vi "Compute Transform Matrix.vi"() -> (0 "Inverse Matrix":T2 format="%.3g", 1 "Beam Angle Deg":dbl[](array[numeric]), 2 "Calibration Factor m/s per MHz":dbl[](array[numeric]) format="%#.3f", 3 "Beam Separations":dbl[](array[numeric]) format="%#.3g", 4 "Meas Setup File":string, 5 "Fixed Axis":T1(ring))   [LabVIEW 2020]
uses:
  <vilib>/Analysis/Matrix/Datatypes/RealMatrix.ctl
  <vilib>/Analysis/baseanly.llb/Matrix Type of Inverse Matrix.ctl
  Globals/Meas_global.vi
  Globals/Constants_global.vi
  <vilib>/Analysis/baseanly.llb/Real Inverse Matrix.vi
  <vilib>/Analysis/NI_AALBase.lvlib
  <vilib>/Analysis/Matrix/NI_Matrix.lvlib
panel:
  out "Input array":dbl[][](array[numeric])
  out "Location when at Focal Point":dbl[](array[numeric])
  out "Beam Check Positions":dbl[][](array[numeric])
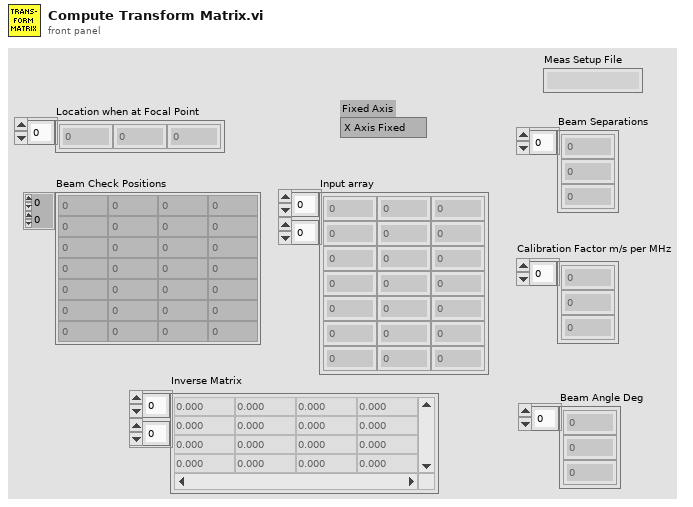
[diagram p1: front panel]
types:
  T1 = enum16{"X Axis Fixed", "Y Axis Fixed", "Z Axis Fixed"}
  T2 = typedef "NI_Matrix.lvlib/RealMatrix.ctl" = dbl[][]
  T3 = typedef "Post_Process.ctl" = enum16{"Take New Data", "Post Process Raw Data File"}
  T4 = typedef "NI_AALBase.lvlib/Matrix Type of Inverse Matrix.ctl" = enum32{"General", "Positive Definite", "Lower Triangular", "Upper Triangular"}
  T5 = typedef "Fixed Axis.ctl" = enum16{"X Axis Fixed", "Y Axis Fixed", "Z Axis Fixed"}
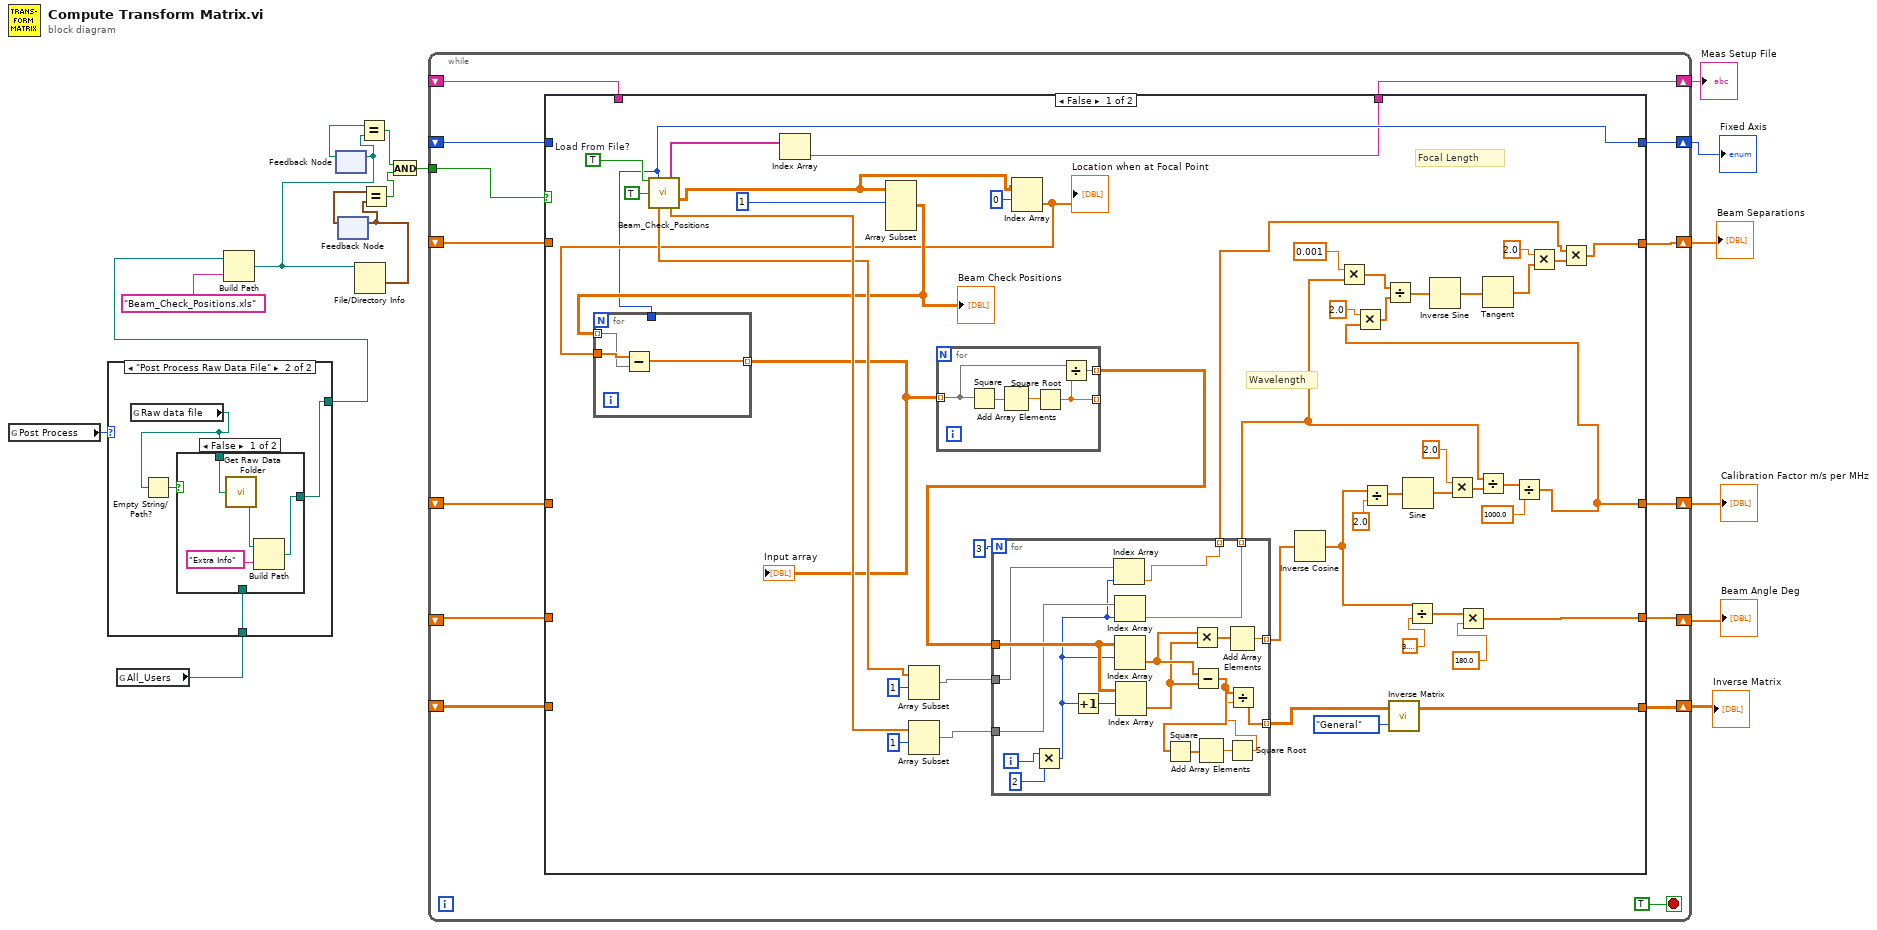
[diagram p0: block diagram]
diagram:
  n1 = global read "Meas_global.vi" "Post Process"() -> (w15:T3)
  n2 = global read "Constants_global.vi" "All_Users"() -> (w7:path)
  n3 = case shown="\"Post Process Raw Data File\"" w15 {
    tunnel: [w18 w22] -> w13
    tunnel: w7 -> [w18 w19]
    frame "Take New Data" {
    }
    frame "Post Process Raw Data File" {
      n4 = global read "Meas_global.vi" "Raw data file"() -> (w21:path)
      n5 = Empty String/Path?(string/path=w21) -> (empty?=w20:bool)
      n6 = case shown="False" w20 {
        tunnel: [w26 w27] -> w22
        tunnel: w21 -> [w24 _]
        tunnel: w19 -> [_ w27]
        frame False {
          n7 = call "Get Raw Data Folder.vi"("Raw data file"=w24) -> ("Main Raw Data Folder"=w23:path)
          n8 = Build Path(base path=w23, name or relative path="Extra Info") -> (appended path=w26:path)
        }
        frame True {
        }
      }
    }
  }
  n9 = Build Path(base path=w13, name or relative path="Beam_Check_Positions.xls" ("Substring")) -> (appended path=w5:path)
  n10 = feedback #1() -> (w4:path)  [unwired: 1 in]
  n11 = feedback-in #1(w5) -> ()
  n12 = feedback #2() -> (w17:timestamp)  [unwired: 1 in]
  n13 = File/Directory Info(path=w5) -> (last mod=w16:timestamp)  [unwired: 1 in, 6 out]
  n14 = feedback-in #2(w16) -> ()
  n15 = Equal?(x=w4, y=w5) -> (x = y?=w2:bool)
  n16 = Equal?(x=w17, y=w16) -> (x = y?=w3:bool)
  n17 = And(x=w2, y=w3) -> (x .and. y?=w1:bool)
  n18 = while {
    tunnel: w1 -> [w32]
    shift-right: [w40] -> w12
    shift-left: _ -> [w39]
    shift-right: [w36] -> w9
    shift-left: _ -> [w35]
    shift-right: [w37] -> w10
    shift-left: _ -> [w34]
    shift-right: [w38] -> w11
    shift-left: _ -> [w33]
    shift-right: [w31] -> w8
    shift-left: _ -> [w30]
    shift-right: [w29] -> w6
    shift-left: _ -> [w28]
    stop <- TRUE stop-if-true
    n19 = case shown="False" w32 {
      tunnel: [w89 w121] -> w40
      tunnel: w39 -> [_ w121]
      tunnel: [w50 w118] -> w38
      tunnel: [w49 w119] -> w37
      tunnel: [w48 w120] -> w36
      tunnel: w35 -> [_ w120]
      tunnel: w34 -> [_ w119]
      tunnel: w33 -> [_ w118]
      tunnel: [w44 w117] -> w31
      tunnel: w30 -> [_ w117]
      tunnel: [w42 w116] -> w29
      tunnel: w28 -> [_ w116]
      frame False {
        w80 = TRUE  # Load From File?
        # "Focal Length"
        # "Wavelength"
        n20 = call "Beam_Check_Positions.vi"("Load From File?"=w80, "Give Focal Point Info (F)"=TRUE) -> ("Fixed Axis"=w44:T5, "Setup File"=w43:string[], "Primary Beam Positions"=w77:dbl[][], "Focal Length"=w54:dbl[], "Wavelength (nm)"=w70:dbl[])  [unwired: 5 in, 4 out]
        n21 = Index Array(array=w43) -> (element=w42:string)  [unwired: 1 in]
        n22 = Array Subset(array=w77, index (row)=1 ("index")) -> (w47:dbl[][])  [unwired: 3 in]
        "Beam Check Positions" <- w47
        n23 = Array Subset(array=w54, index=1) -> (w53:dbl[])  [unwired: 1 in]
        n24 = Array Subset(array=w70, index=1) -> (w68:dbl[])  [unwired: 1 in]
        n25 = Index Array(array=w77, index (row)=0) -> (element=w46:dbl[])  [unwired: 1 in]
        "Location when at Focal Point" <- w46
        n26 = for {
          tunnel: w47 -> [w91] mode=indexing
          tunnel: w46 -> [w92]
          tunnel: w44 -> [_]
          tunnel: [w90] -> w45 mode=indexing
          n27 = Subtract(x=w92, y=w91) -> (x-y=w90:dbl[])
        }
        "Input array" <- w45
        n28 = for {
          tunnel: w45 -> [w112] mode=indexing
          tunnel: [w113] -> _ mode=indexing
          tunnel: [w111] -> w87 mode=indexing
          n29 = Square(x=w112) -> (x^2=w115:dbl[])
          n30 = Add Array Elements(numeric array=w115) -> (sum=w114:dbl)
          n31 = Square Root(x=w114) -> (sqrt(x)=w113:dbl)
          n32 = Divide(x=w112, y=w113) -> (x/y=w111:dbl[])
        }
        n33 = for {
          N: 3 -> [_]
          tunnel: w87 -> [w108]
          tunnel: [w105] -> w86 mode=indexing
          tunnel: [w100] -> w82 mode=indexing
          tunnel: w68 -> [w97]
          tunnel: [w96] -> w63 mode=indexing
          tunnel: w53 -> [w94]
          tunnel: [w93] -> w51 mode=indexing
          i -> [w110]
          n34 = Multiply(x=w110, y=2) -> (x*y=w95:i32)
          n35 = Increment(x=w95) -> (x+1=w107:i32)
          n36 = Index Array(array=w94, index=w95) -> (element=w93:dbl)
          n37 = Index Array(array=w97, index=w95) -> (element=w96:dbl)
          n38 = Index Array(array=w108, index (row)=w95) -> (element=w104:dbl[])  [unwired: 1 in]
          n39 = Index Array(array=w108, index (row)=w107) -> (element=w103:dbl[])  [unwired: 1 in]
          n40 = Multiply(x=w104, y=w103) -> (x*y=w106:dbl[])
          n41 = Subtract(x=w104, y=w103) -> (x-y=w99:dbl[])
          n42 = Square(x=w99) -> (x^2=w102:dbl[])
          n43 = Add Array Elements(numeric array=w102) -> (sum=w101:dbl)
          n44 = Add Array Elements(numeric array=w106) -> (sum=w105:dbl)
          n45 = Square Root(x=w101) -> (sqrt(x)=w98:dbl)
          n46 = Divide(x=w99, y=w98) -> (x/y=w100:dbl[])
        }
        n47 = Inverse Cosine(1:w86) -> (0:w75:dbl[])
        n48 = Multiply(x=0.001, y=w63) -> (x*y=w61:dbl[])
        n49 = Divide(x=w75, y=2.0) -> (x/y=w73:dbl[])
        n50 = call-poly <vilib>:"Inverse Matrix.vi"("matrix type"=Matrix_Type_of_Inverse_Matrix."General", "Input Matrix"=w82) -> ("Inverse Matrix"=w89:T2)  [unwired: 1 out]
        n51 = Sine(x=w73) -> (sin(x)=w72:dbl[])
        n52 = Divide(x=w75, y=3.141592653589793) -> (x/y=w84:dbl[])
        n53 = Multiply(x=2.0, y=w72) -> (x*y=w67:dbl[])
        n54 = Multiply(x=w84, y=180.0) -> (x*y=w50:dbl[])
        n55 = Divide(x=w63, y=w67) -> (x/y=w66:dbl[])
        n56 = Divide(x=w66, y=1000.0) -> (x/y=w49:dbl[])
        n57 = Multiply(x=2.0, y=w49) -> (x*y=w60:dbl[])
        n58 = Divide(x=w61, y=w60) -> (x/y=w59:dbl[])
        n59 = Inverse Sine(1:w59) -> (0:w57:dbl[])
        n60 = Tangent(1:w57) -> (0:w56:dbl[])
        n61 = Multiply(x=2.0, y=w56) -> (x*y=w52:dbl[])
        n62 = Multiply(x=w51, y=w52) -> (x*y=w48:dbl[])
      }
      frame True {
      }
    }
  }
  "Inverse Matrix" <- w12
  "Beam Angle Deg" <- w11
  "Calibration Factor m/s per MHz" <- w10
  "Beam Separations" <- w9
  "Fixed Axis" <- w8
  "Meas Setup File" <- w6
